vi "Tosca-Clean Up AI Processing.vi"(0 "state":T1) -> ()   [LabVIEW 2020]
uses:
  Typedefs/Tosca-AI Plot State.ctl
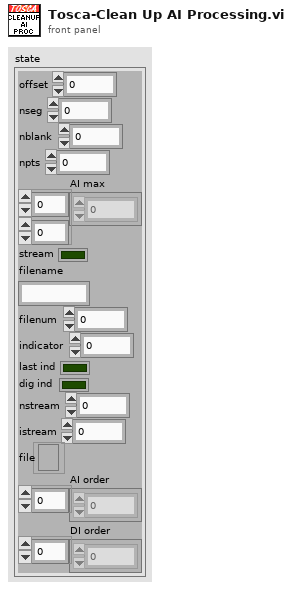
[diagram p1: front panel]
types:
  T1 = typedef "Tosca-AI Plot State.ctl" = cluster{"offset":i32, "nseg":i32, "nblank":i32, "npts":i32, "AI max":dbl[][], "stream":bool, "filename":string, "filenum":i32, "indicator":i32, "last ind":bool, "dig ind":bool, "nstream":i32, "istream":i32, "file":refnum<file>, "AI order":i32[], "DI order":i32[]}
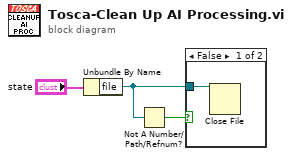
[diagram p0: block diagram]
diagram:
  n1 = Unbundle By Name("state") -> ("file"=w2:refnum<file>)
  n2 = Not A Number/Path/Refnum?(number/path/refnum=w2) -> (NaN/Path/Refnum?=w1:bool)
  n3 = case shown="False" w1 {
    tunnel: w2 -> [w4 _]
    frame False {
      n4 = Close File(refnum=w4) -> ()  [unwired: 1 in, 2 out]
    }
    frame True {
    }
  }
